vi "GPS-SCADA.vi"() -> ()   [LabVIEW 2022 SP3]
panel:
  out "Segundo Dato : Tiempo UTC":string
  out "Longitud Procesada":dbl
  out "Latitud Procesada":dbl
  out "Señal del GPS":bool
  out "Treceavo Dato":string
  out "Deceavo Dato":string
  out "Octavo Dato : Fix":string
  out "Noveno : Satelites en Seguimiento":string
  out "Decimo Dato":string
  out "Onceavo Dato":string
  out "Setimo Dato : E/w":string
  out "Sexto Dato":string
  out "Quinto Dato : Longitud":string
  out "Tercer Dato : Latitud":string
  out "Cuarto Dato : N/S":string
  out "Segundo Dato : Tiempo UTC-5-Peru-Procesada":string
  out "Primer Dato: Tipo de trama gps":string
  out "Dato GPGGA":bool
  out "Dato de Comparacion":string
  in  "Control":bool
  in  "Trama Recibida del GPS":string
  # "Dato de Prueba: $GPGGA,123519,4807.038,N,01131,000,E,2,08,0.9,545.4,M,46.9,M,,*42"
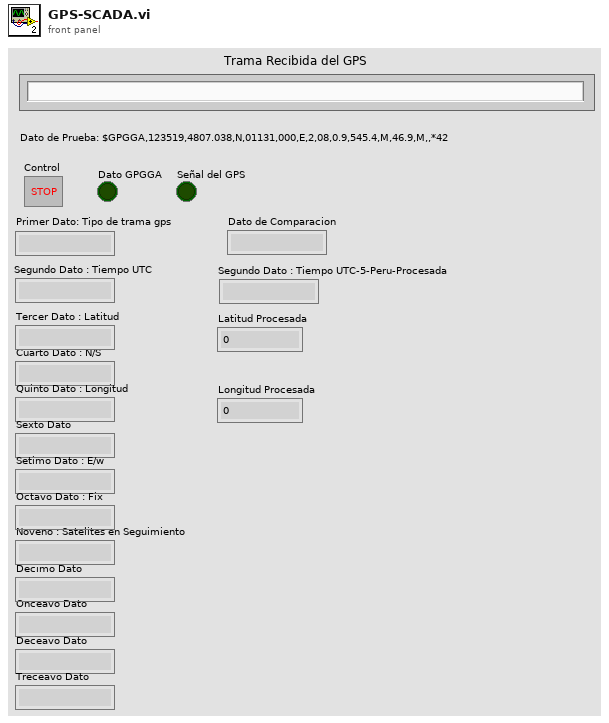
[diagram p1: front panel]
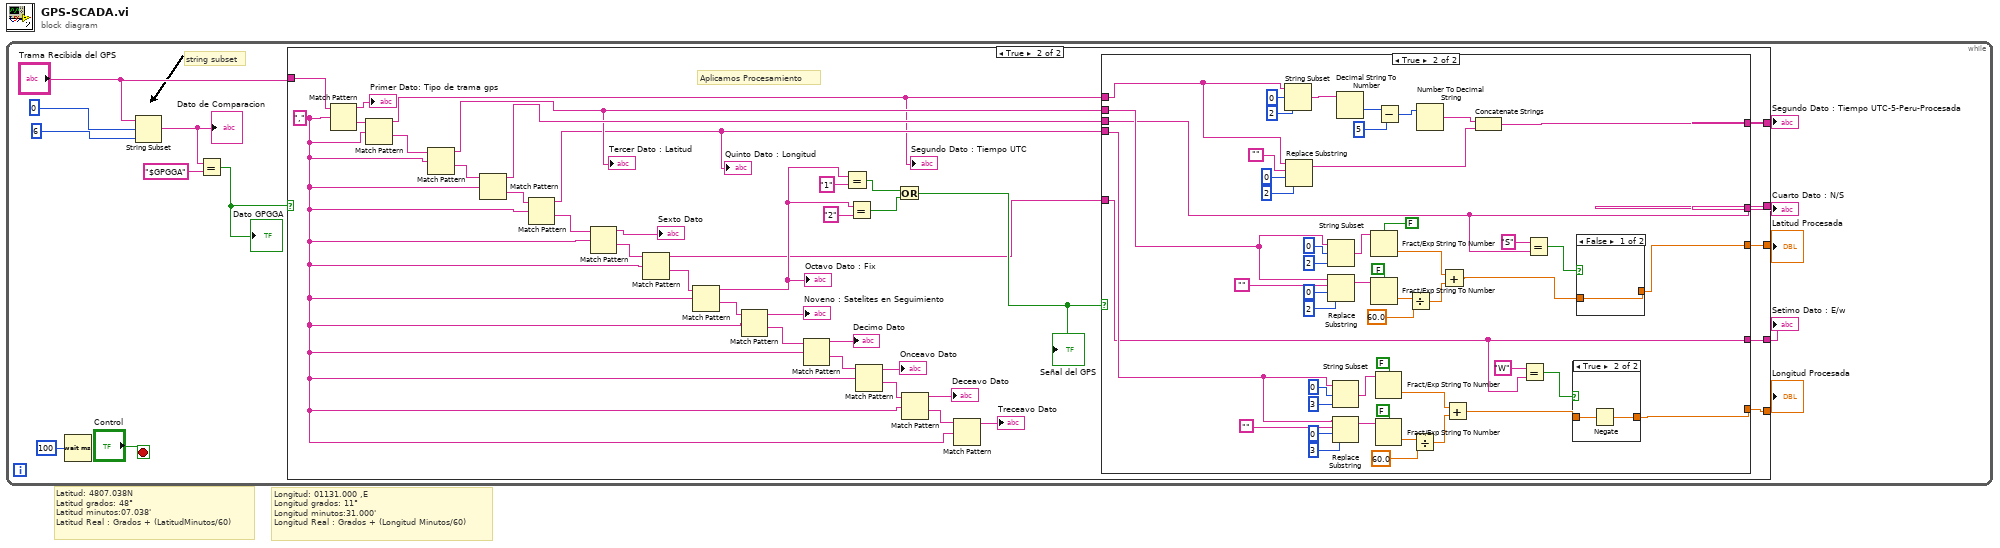
[diagram p0: block diagram]
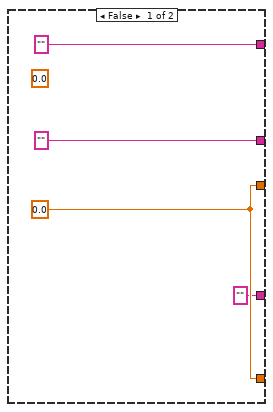
[diagram p2: hidden frame]
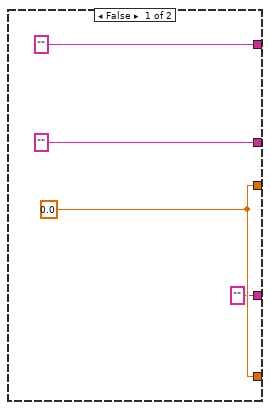
[diagram p3: hidden frame]
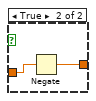
[diagram p5: hidden frame]
diagram:
  # "Longitud: 01131.000 ,E\nLongitud grados: 11°\nLongitud minutos:31.000'\nLongitud Real : Grados + (Longitud Minutos/60)"
  # "Latitud: 4807.038N\nLatitud grados: 48°\nLatitud minutos:07.038'\nLatitud Real : Grados + (LatitudMinutos/60)"
  n1 = while {
    stop <- "Control" stop-if-true
    # "string subset"
    n2 = Wait (ms)(milliseconds to wait=u32 100) -> ()  [unwired: 1 out]
    n3 = String Subset(string="Trama Recibida del GPS", offset (0)=0, length (rest)=6 ("length (rest)")) -> (substring=w9:string)
    "Dato de Comparacion" <- w9
    n4 = Equal?(x=w9, y="$GPGGA") -> (x = y?=w7:bool)
    "Dato GPGGA" <- w7
    n5 = case shown="True" w7 {
      tunnel: "Trama Recibida del GPS" -> [_ w54]
      tunnel: ["" w28] -> w5
      tunnel: ["" ("Trama Recibida del GPS") w27] -> w4
      tunnel: ["" ("Trama Recibida del GPS") w20] -> w3
      tunnel: [w15 w19] -> w2
      tunnel: [w15 w18] -> w1
      frame False {
        w15 = 0.0
        (unwired) 0.0
      }
      frame True {
        w37 = "," ("regular expression")
        # "Aplicamos Procesamiento"
        n6 = Match Pattern(string=w54, regular expression=w37) -> (before substring=→"Primer Dato: Tipo de trama gps":string, after substring=w53:string)  [unwired: 1 in, 2 out]
        n7 = Match Pattern(string=w53, regular expression=w37) -> (before substring=w22:string, after substring=w52:string)  [unwired: 1 in, 2 out]
        "Segundo Dato : Tiempo UTC" <- w22
        n8 = Match Pattern(string=w52, regular expression=w37) -> (before substring=w26:string, after substring=w51:string)  [unwired: 1 in, 2 out]
        "Tercer Dato : Latitud" <- w26
        n9 = Match Pattern(string=w51, regular expression=w37) -> (before substring=w31:string, after substring=w48:string)  [unwired: 1 in, 2 out]
        n10 = Match Pattern(string=w48, regular expression=w37) -> (before substring=w25:string, after substring=w50:string)  [unwired: 1 in, 2 out]
        "Quinto Dato : Longitud" <- w25
        n11 = Match Pattern(string=w50, regular expression=w37) -> (before substring=→"Sexto Dato":string, after substring=w49:string)  [unwired: 1 in, 2 out]
        n12 = Match Pattern(string=w49, regular expression=w37) -> (before substring=w21:string, after substring=w42:string)  [unwired: 1 in, 2 out]
        n13 = Match Pattern(string=w42, regular expression=w37) -> (before substring=w23:string, after substring=w29:string)  [unwired: 1 in, 2 out]
        "Octavo Dato : Fix" <- w23
        n14 = Match Pattern(string=w29, regular expression=w37) -> (before substring=→"Noveno : Satelites en Seguimiento":string, after substring=w43:string)  [unwired: 1 in, 2 out]
        n15 = Match Pattern(string=w43, regular expression=w37) -> (before substring=→"Decimo Dato":string, after substring=w44:string)  [unwired: 1 in, 2 out]
        n16 = Equal?(x=w23, y="1") -> (x = y?=w34:bool)
        n17 = Equal?(x=w23, y="2") -> (x = y?=w33:bool)
        n18 = Match Pattern(string=w44, regular expression=w37) -> (before substring=→"Onceavo Dato":string, after substring=w38:string)  [unwired: 1 in, 2 out]
        n19 = Or(x=w34, y=w33) -> (x .or. y?=w32:bool)
        "Señal del GPS" <- w32
        n20 = Match Pattern(string=w38, regular expression=w37) -> (before substring=→"Deceavo Dato":string, after substring=w39:string)  [unwired: 1 in, 2 out]
        n21 = Match Pattern(string=w39, regular expression=w37) -> (before substring=→"Treceavo Dato":string)  [unwired: 1 in, 3 out]
        n22 = case shown="True" w32 {
          tunnel: w22 -> [_ w72]
          tunnel: w26 -> [_ w83]
          tunnel: w31 -> [_ w68]
          tunnel: w25 -> [_ w82]
          tunnel: ["" w69] -> w28
          tunnel: ["" ("Trama Recibida del GPS") w68] -> w27
          tunnel: w21 -> [_ w59]
          tunnel: ["" ("Trama Recibida del GPS") w59] -> w20
          tunnel: [w56 w64] -> w19
          tunnel: [w56 w60] -> w18
          frame False {
            w56 = 0.0
          }
          frame True {
            n23 = String Subset(string=w72, offset (0)=0, length (rest)=2 ("length (rest)")) -> (substring=w79:string)
            n24 = Replace Substring(2:2 ("length (len. of substring)"), 3:0 ("offset (0)"), 4:"", 5:w72) -> (1:w70:string)  [unwired: 1 out]
            n25 = String Subset(string=w83, offset (0)=0, length (rest)=2 ("length (rest)")) -> (substring=w104:string)
            n26 = Replace Substring(2:2 ("length (len. of substring)"), 3:0 ("offset (0)"), 4:"", 5:w83) -> (1:w103:string)  [unwired: 1 out]
            n27 = String Subset(string=w82, offset (0)=0, length (rest)=3 ("length (rest)")) -> (substring=w91:string)
            n28 = Replace Substring(2:3 ("length (len. of substring)"), 3:0 ("offset (0)"), 4:"", 5:w82) -> (1:w90:string)  [unwired: 1 out]
            n29 = Decimal String To Number(string=w79) -> (number=w78:i32)  [unwired: 2 in, 1 out]
            n30 = Fract/Exp String To Number(use system decimal point (T)=FALSE, string=w104) -> (number=w100:dbl)  [unwired: 2 in, 1 out]
            n31 = Fract/Exp String To Number(use system decimal point (T)=FALSE, string=w103) -> (number=w102:dbl)  [unwired: 2 in, 1 out]
            n32 = Fract/Exp String To Number(use system decimal point (T)=FALSE, string=w91) -> (number=w87:dbl)  [unwired: 2 in, 1 out]
            n33 = Fract/Exp String To Number(use system decimal point (T)=FALSE, string=w90) -> (number=w89:dbl)  [unwired: 2 in, 1 out]
            n34 = Subtract(x=w78, y=5) -> (x-y=w76:i32)
            n35 = Divide(x=w102, y=60.0) -> (x/y=w99:dbl)
            n36 = Divide(x=w89, y=60.0) -> (x/y=w86:dbl)
            n37 = Number To Decimal String(number=w76) -> (decimal integer string=w71:string)  [unwired: 1 in]
            n38 = Add(x=w100, y=w99) -> (x+y=w65:dbl)
            n39 = Add(x=w87, y=w86) -> (x+y=w61:dbl)
            n40 = Concatenate Strings(w71, w70) -> (w69:string)
            n41 = Equal?(x="W", y=w59) -> (x = y?=w63:bool)
            n42 = Equal?(x="S", y=w68) -> (x = y?=w66:bool)
            n43 = case shown="True" w63 {
              tunnel: [w110 w112] -> w60
              tunnel: w61 -> [w110 w111]
              frame False {
              }
              frame True {
                n44 = Negate(x=w111) -> (-x=w112:dbl)
              }
            }
            n45 = case shown="False" w66 {
              tunnel: w65 -> [w113 w115]
              tunnel: [w113 w114] -> w64
              frame False {
              }
              frame True {
                n46 = Negate(x=w115) -> (-x=w114:dbl)
              }
            }
          }
        }
      }
    }
    "Latitud Procesada" <- w2
    "Longitud Procesada" <- w1
    "Segundo Dato : Tiempo UTC-5-Peru-Procesada" <- w5
    "Cuarto Dato : N/S" <- w4
    "Setimo Dato : E/w" <- w3
  }
